vi "Migration Energy Script.vi"() -> ()   [LabVIEW 2010]
panel:
  in  "Folder Name":string
  in  "New Directory":path=path "D:/Ab-initio/VASP Calcs/2D_Grain Boundaries/Batch38_20130927"
  in  "2nd POSCAR":path
  in  "1st POSCAR":path
  in  "# Frames":i32=5
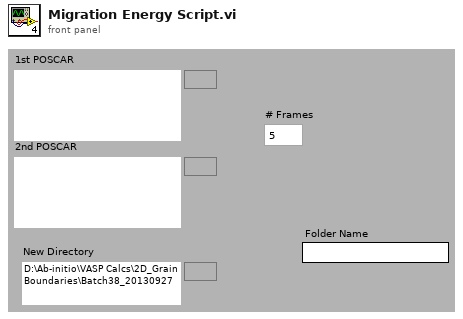
[diagram p1: front panel]
types:
  T1 = cluster{"Structure Name":string, "Lattice vector a":dbl[], "Lattice vector b":dbl[], "Lattice vector c":dbl[], "Atoms Array":cluster{"Atom Name":string, "Positions (Direct)":dbl[][], "Positions (Cartesian)":dbl[][]}[], "# of atoms":i32}
  T2 = cluster{"Structure Name":string, "Lattice vector a":dbl[], "Lattice vector b":dbl[], "Lattice vector c":dbl[], "Atoms Array":cluster{"Atom Name":string, "Positions (Direct)":dbl[][], "Positions (Cartesian)":dbl[][]}[], "# of atoms":i32}[]
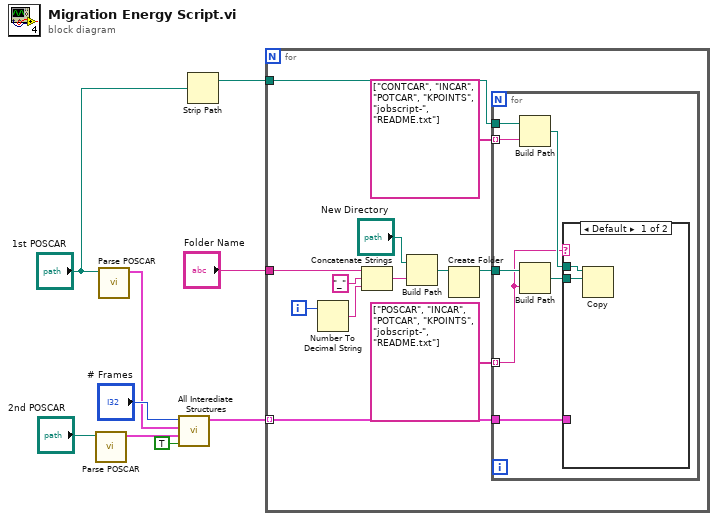
[diagram p0: block diagram]
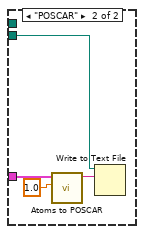
[diagram p2: hidden frame]
diagram:
  n1 = call "Parse POSCAR.vi"("POSCAR File"="2nd POSCAR") -> ("Structure"=w8:T1)  [unwired: 7 in, 3 out]
  n2 = call "Parse POSCAR.vi"("POSCAR File"="1st POSCAR") -> ("Structure"=w6:T1)  [unwired: 7 in, 3 out]
  n3 = call "All Interediate Structures.vi"("Map back to [0,1) ?"=TRUE, "Second Structure"=w8, "First Structure"=w6, "# Frames"="# Frames") -> ("Array of Structures"=w5:T2)  [unwired: 7 in]
  n4 = Strip Path(path="1st POSCAR") -> (stripped path=w3:path)  [unwired: 1 out]
  n5 = for {
    tunnel: w3 -> [w10]
    tunnel: "Folder Name" -> [w14]
    tunnel: w5 -> [w11] mode=indexing
    i -> [w13]
    n6 = Number To Decimal String(number=w13) -> (decimal integer string=w15:string)  [unwired: 1 in]
    n7 = Concatenate Strings(w14, "_" ("string"), w15) -> (w16:string)
    n8 = Build Path(base path="New Directory", name or relative path=w16) -> (appended path=w20:path)
    n9 = Create Folder(path (use dialog)=w20) -> (created path=w19:path)  [unwired: 2 in, 2 out]
    n10 = for {
      tunnel: w10 -> [w28]
      tunnel: w19 -> [w25]
      tunnel: string[] ["CONTCAR", "INCAR", "POTCAR", "KPOINTS", "jobscript-", "README.txt"] -> [w27] mode=indexing
      tunnel: string[] ["POSCAR", "INCAR", "POTCAR", "KPOINTS", "jobscript-", "README.txt"] -> [w23] mode=indexing
      tunnel: w11 -> [w22]
      n11 = Build Path(base path=w28, name or relative path=w27) -> (appended path=w26:path)
      n12 = Build Path(base path=w25, name or relative path=w23) -> (appended path=w24:path)
      n13 = case shown="Default" w23 {
        tunnel: w26 -> [w30 _]
        tunnel: w24 -> [w29 w31]
        tunnel: w22 -> [_ w33]
        frame Default {
          n14 = Copy(10:w29, 11:w30) -> ()  [unwired: 3 in, 3 out]
        }
        frame "POSCAR" {
          n15 = call "Atoms to POSCAR.vi"("Volume Factor"=1.0, "Atomic Structure"=w33) -> ("POSCAR File"=w34:string)  [unwired: 9 in]
          n16 = Write to Text File(file (use dialog)=w31, text=w34) -> ()  [unwired: 2 in, 3 out]
        }
      }
    }
  }
